vi "beginSimplePassPlay.vi"(8 "error in (no error)":errorcluster, 9 "last command_interpreted":T1, 10 "Game in":refnum<class "Game.lvclass">, 11 "SimplePass in":refnum<class "SimplePass.lvclass">) -> (0 "error out":errorcluster, 2 "BeginSimplePass?":bool, 3 "SimplePass out":refnum<class "SimplePass.lvclass">)   [LabVIEW 2023, in "SimplePass.lvclass"]
uses:
  SimplePass.lvclass
  Game_class/Game.lvclass
  Referee_class/command_interpreted.ctl
  Game_class/Game.lvclass/Game.ctl
  Referee_class/Referee.lvclass/Referee.ctl
  Parameters_class/Parameters.lvclass/Parameters.ctl
  Game_class/Read Referee.vi
  Game_class/Read Parameters.lvclass.vi
  Parameters_class/Read SimplePass.vi
  Referee_class/Read command_interpreted.vi
  Referee_class/Referee.lvclass
  Parameters_class/Parameters.lvclass
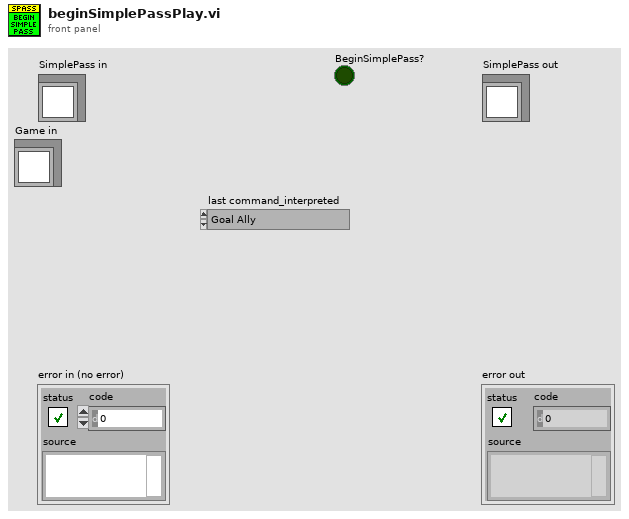
[diagram p1: front panel]
types:
  T1 = typedef "command_interpreted.ctl" = enum16{"Goal Ally", "Goal Enemy", "Ball Placement Enemy", "Ball Placement Ally", "Normal Half Time", "Extra Time  Break", "Extra Half Time", "None", "Post Game", "PKA Normal Start", "Prepare Kickoff Ally", "PKE Normal Start", "Prepare Kickoff Enemy", "Force Start", "Halt", "Timeout", "Prepare Penalty Ally", "Prepare Penalty Enemy", "PPA NormalStart", "PPE Normal Start", "Indirect Free Ally", "Direct Free Enemy", "Direct Free Ally", "Indirect Free Enemy", "Stop"}
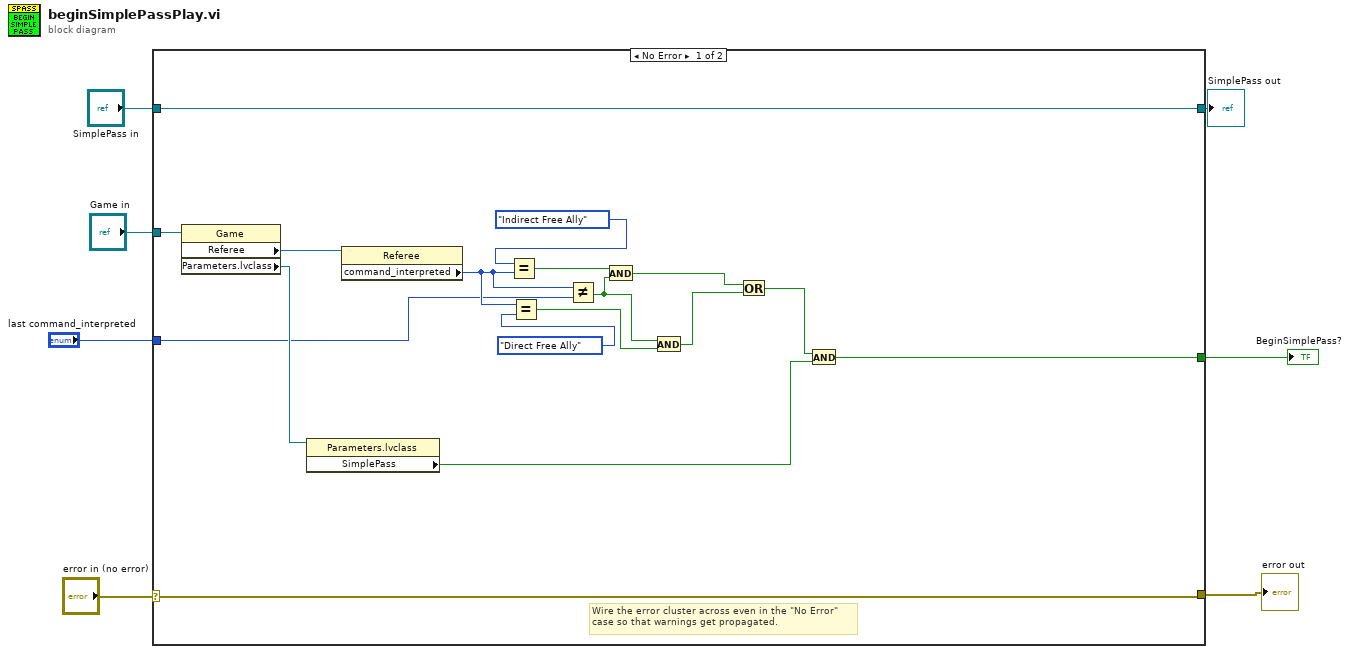
[diagram p0: block diagram]
diagram:
  n1 = case shown="No Error" "error in (no error)" {
    selector: "error in (no error)" -> [w24 w26]
    tunnel: [w24 w26] -> w6
    tunnel: [w11 w25] -> w4
    tunnel: "SimplePass in" -> [w11 w25]
    tunnel: "Game in" -> [w23 _]
    tunnel: [w12 _] -> w2
    tunnel: "last command_interpreted" -> [w8 _]
    frame No Error {
      # "Wire the error cluster across even in the \"No Error\"\ncase so that warnings get propagated."
      n2 = property class="Game"(reference=w23) -> ("Referee"=w22:refnum<class "Referee.lvclass">, "Parameters.lvclass"=w10:refnum<class "Parameters.lvclass">)  [unwired: 1 in, 2 out]
      n3 = property class="Parameters.lvclass"(reference=w10) -> ("SimplePass"=w9:bool)  [unwired: 1 in, 2 out]
      n4 = property class="Referee"(reference=w22) -> ("command_interpreted"=w15:T1)  [unwired: 1 in, 2 out]
      n5 = Equal?(x=command_interpreted."Indirect Free Ally" ("command_interpreted"), y=w15) -> (x = y?=w21:bool)
      n6 = Equal?(x=w15, y=command_interpreted."Direct Free Ally" ("command_interpreted")) -> (x = y?=w17:bool)
      n7 = Not Equal?(x=w15, y=w8) -> (x != y?=w14:bool)
      n8 = And(x=w21, y=w14) -> (x .and. y?=w19:bool)
      n9 = And(x=w14, y=w17) -> (x .and. y?=w16:bool)
      n10 = Or(x=w19, y=w16) -> (x .or. y?=w13:bool)
      n11 = And(x=w13, y=w9) -> (x .and. y?=w12:bool)
    }
    frame Error {
    }
  }
  "error out" <- w6
  "SimplePass out" <- w4
  "BeginSimplePass?" <- w2
